vi "punto_2 - copia.vi"() -> ()   [LabVIEW 2019]
panel:
  in  "Acción":bool
  in  "Llenado/Vaciado":bool
  in  "Velocidad":bool
  out "Tanque Vacio":bool
  out "Tanque Lleno":bool
  out "Paro":bool
  out "Llenando":bool
  out "Vaciando":bool
  out "Tanque":dbl(slide) scale=0.0..1000.0
  # "Alta"
  # "Baja"
  # "continuar"
  # "Parar"
  # "Llenar"
  # "Vaciar"
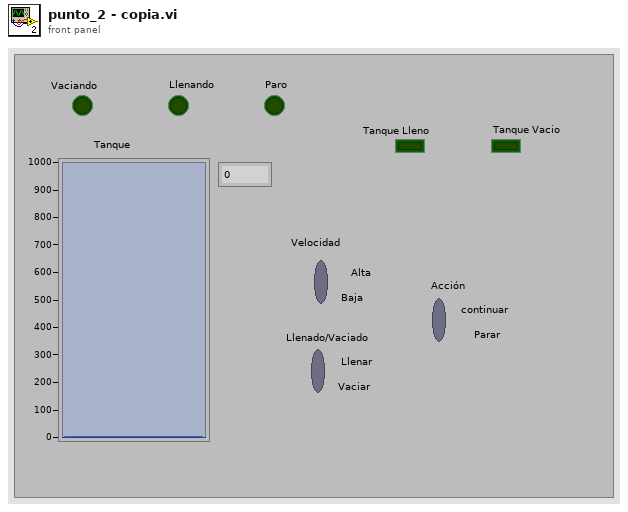
[diagram p1: front panel]
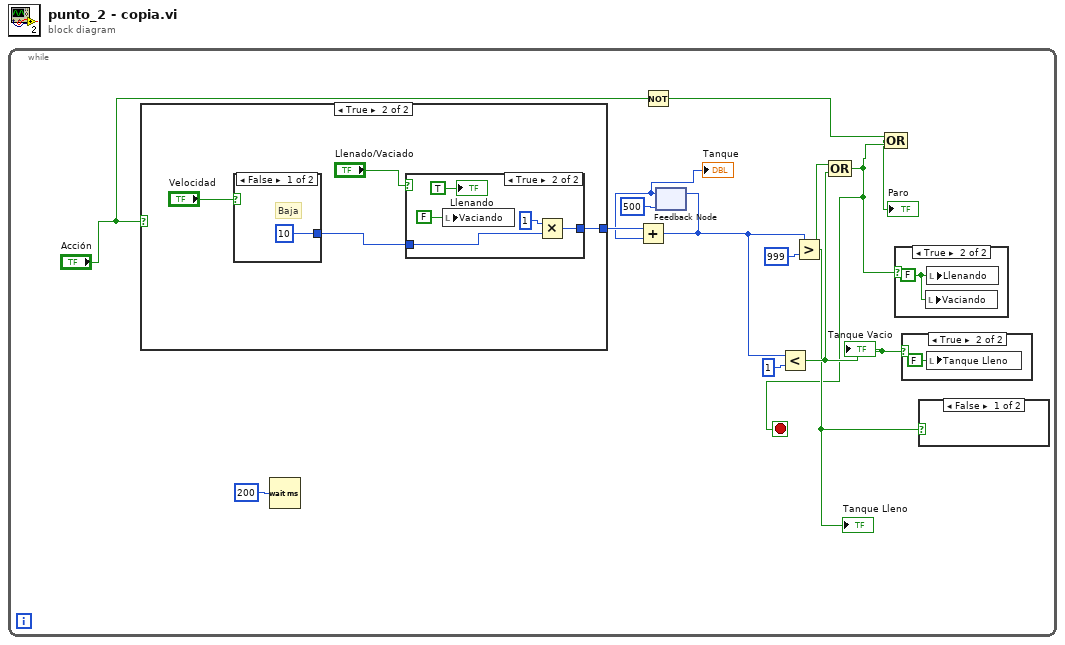
[diagram p0: block diagram]
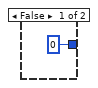
[diagram p2: hidden frame]
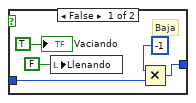
[diagram p3: hidden frame]
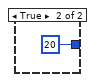
[diagram p4: hidden frame]
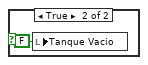
[diagram p5: hidden frame]
diagram:
  n1 = while {
    stop <- w3 stop-if-true
    n2 = case shown="True" "Acción" {
      tunnel: [0 w15] -> w11
      frame False {
      }
      frame True {
        n3 = case shown="False" "Velocidad" {
          tunnel: [10 20] -> w17
          frame False {
            # "Baja"
          }
          frame True {
          }
        }
        n4 = case shown="True" "Llenado/Vaciado" {
          tunnel: w17 -> [w22 w28]
          tunnel: [w21 w26] -> w15
          frame False {
            # "Baja"
            n5 = local write "Llenando"(FALSE ("Llenando")) -> ()
            n6 = Multiply(x=-1, y=w22) -> (x*y=w21:i32)
            "Vaciando" <- TRUE ("Vaciando")
          }
          frame True {
            n7 = local write "Vaciando"(FALSE ("Vaciando")) -> ()
            n8 = Multiply(x=1 ("y"), y=w28) -> (x*y=w26:i32)
            "Llenando" <- TRUE ("Llenando")
          }
        }
      }
    }
    n9 = Wait (ms)(milliseconds to wait=u32 200) -> ()  [unwired: 1 out]
    n10 = Not(x="Acción") -> (.not. x?=w2:bool)
    n11 = feedback #1(500) -> (w8:i32)
    "Tanque" <- w8
    n12 = Add(x=w11, y=w8) -> (x+y=w4:i32)
    n13 = feedback-in #1(w4) -> ()
    n14 = Less?(x=w4, y=1) -> (x < y?=w7:bool)
    "Tanque Vacio" <- w7
    n15 = Greater?(x=w4, y=999) -> (0:w5:bool)
    "Tanque Lleno" <- w5
    n16 = Compound Arithmetic op=OR(w5, w7) -> (w3:bool)
    n17 = Compound Arithmetic op=OR(w2, w3) -> (→"Paro":bool)
    n18 = case shown="True" w3 {
      frame False {
      }
      frame True {
        w33 = FALSE ("Llenando")
        n19 = local write "Vaciando"(w33) -> ()
        n20 = local write "Llenando"(w33) -> ()
      }
    }
    n21 = case shown="True" w7 {
      frame False {
      }
      frame True {
        n22 = local write "Tanque Lleno"(FALSE ("Llenando")) -> ()
      }
    }
    n23 = case shown="False" w5 {
      frame False {
      }
      frame True {
        n24 = local write "Tanque Vacio"(FALSE ("Tanque Vacio")) -> ()
      }
    }
  }
